vi "Weather_Buffer_Data.vi"(10 "Parsed Data Array":dbl[](array[numeric]), 11 "Un-Parsed String":string) -> (3 "Plot Arrays":dbl[][](array[numeric]))   [LabVIEW 2018]
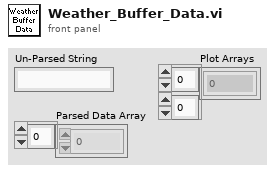
[diagram p1: front panel]
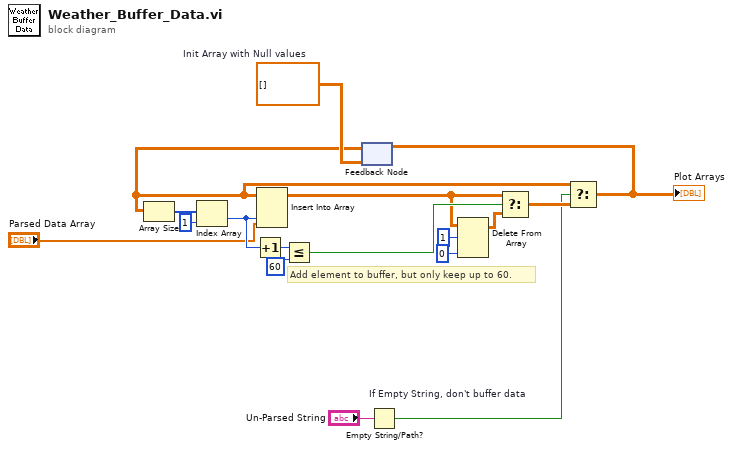
[diagram p0: block diagram]
diagram:
  w17 = dbl[][] []  # Init Array with Null values
  # "Add element to buffer, but only keep up to 60."
  n1 = feedback #1(w17) -> (w2:dbl[][])
  n2 = Array Size(array=w2) -> (size(s)=w7:i32[])
  n3 = Index Array(array=w7, index=1) -> (element=w9:i32)
  n4 = Increment(x=w9) -> (x+1=w10:i32)
  n5 = Insert Into Array(array=w2, index (col)=w9, new element="Parsed Data Array") -> (w5:dbl[][])  [unwired: 1 in]
  n6 = Less Or Equal?(x=w10, y=60) -> (x <= y?=w12:bool)
  n7 = Empty String/Path? "If Empty String, don't buffer data"(string/path="Un-Parsed String") -> (empty?=w1:bool)
  n8 = Delete From Array(array=w5, length=1, index (col)=0 ("disabled index (col)")) -> (array with subset deleted=w13:dbl[][])  [unwired: 1 in, 1 out]
  n9 = Select(t=w5, s=w12, f=w13) -> (s? t:f=w4:dbl[][])
  n10 = Select(t=w2, s=w1, f=w4) -> (s? t:f=w3:dbl[][])
  "Plot Arrays" <- w3
  n11 = feedback-in #1(w3) -> ()
